vi "time course only.vi"() -> ()   [LabVIEW 2016]
uses:
  <vilib>/Utility/file.llb/Read Delimited Spreadsheet (string).vi
  <vilib>/Analysis/NI_AALBase.lvlib
panel:
  out "Histogram Graph 2":T1(graph)
  out "Histogram Graph":T1(graph)
  in  "Save ?":bool
  in  "∮":dbl=4.0
  in  "BM":dbl=23.16
  in  "smooth line":i32=300
  in  "Next Button":bool
  in  "stop 2":dbl=31894.0
  in  "stop":dbl=31744.0
  in  "start 2":dbl=29984.0
  in  "start":dbl=30134.0
  out "XY Graph 2":cluster{dbl[], dbl[]}[](graph)
  out "appended path":path
  out "Filenames":string[](array[string])
  in  "Path Folder":path
  out "path out":path
  out "# of frames":dbl
  out "aoi count repeat":dbl[](array[numeric])
  out "Tandem Yi position":dbl[](array[numeric])
  out "Tandem Xi position":dbl[](array[numeric])
  out "# of AOIs":dbl
  # "Highlight"
  # "Buffer wash"
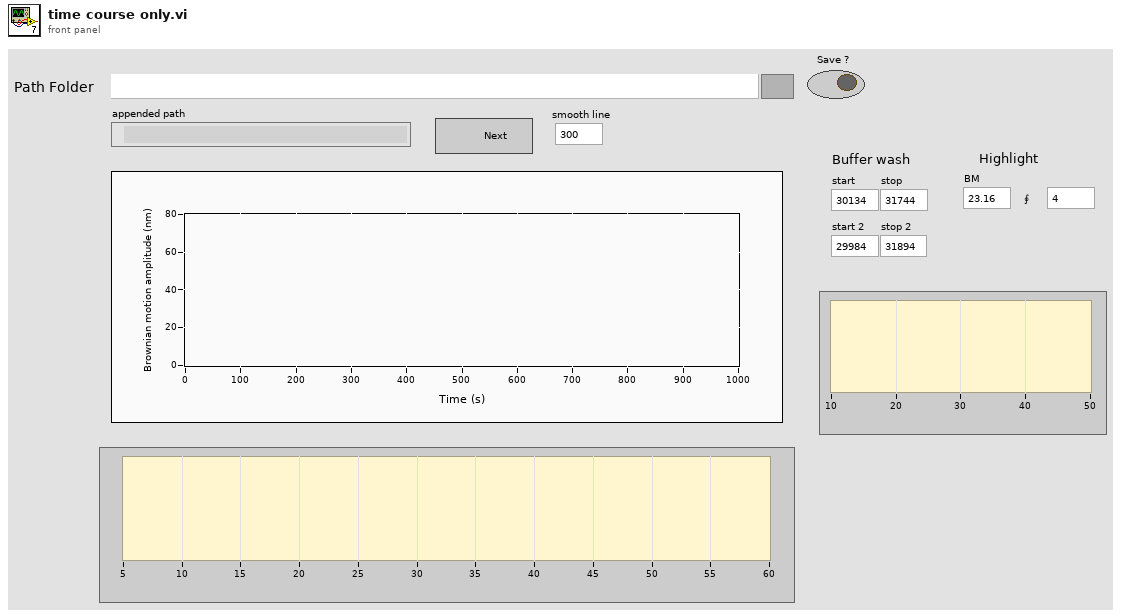
[diagram p1: front panel]
types:
  T1 = cluster{"X Values":dbl[], "Histogram: h(x)":i32[]}
  T2 = typedef "imagedata.ctl" = cluster{"image type":i32, "image depth":i32, "image":u8[], "mask":u8[], "colors":u32[], "Rectangle":cluster{"left":i16, "top":i16, "right":i16, "bottom":i16}}
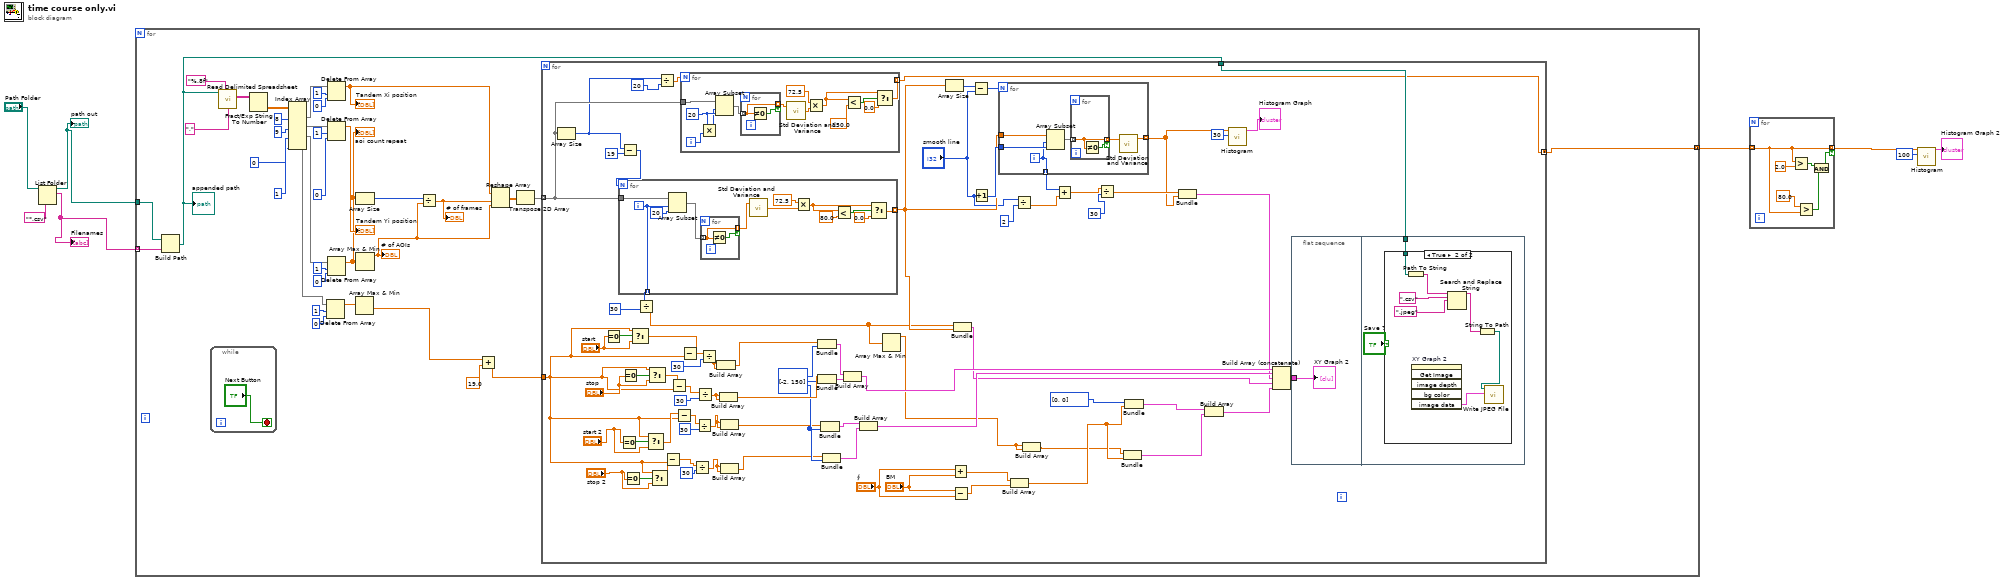
[diagram p0: block diagram]
diagram:
  n1 = List Folder(path="Path Folder", pattern="*.csv") -> (path out=w6:path, filenames=w5:string[])  [unwired: 2 in, 2 out]
  "path out" <- w6
  "Filenames" <- w5
  n2 = for {
    tunnel: w6 -> [w19]
    tunnel: w5 -> [w20] mode=indexing
    tunnel: [w9] -> w2 mode=concatenating
    n3 = Build Path(base path=w19, name or relative path=w20) -> (appended path=w10:path)
    "appended path" <- w10
    n4 = while {
      stop <- "Next Button" stop-if-true
    }
    n5 = call-poly <vilib>:"Read Delimited Spreadsheet.vi"("file path (dialog if empty)"=w10, "format (%s)"="%.8f" ("format (%.3f)"), "delimiter (\\t)"="," ("delimiter (\\t)")) -> ("all rows"=w42:string[][])  [unwired: 7 in, 5 out]
    n6 = Fract/Exp String To Number(string=w42) -> (number=w26:dbl[][])  [unwired: 3 in, 1 out]
    n7 = Index Array(array=w26, index (col) #1=8 ("disabled index (col)"), index (col) #2=9 ("index (col)"), index (col) #3=1 ("index (col)"), index (col) #4=0 ("index (col)")) -> (element #1=w34:dbl[], element #2=w35:dbl[], element #3=w30:dbl[], element #4=w15:dbl[])  [unwired: 4 in]
    n8 = Delete From Array(array=w15, length=1, index=0) -> (array with subset deleted=w14:dbl[])  [unwired: 1 out]
    n9 = Delete From Array(array=w34, length=1, index=0) -> (array with subset deleted=w25:dbl[])  [unwired: 1 out]
    "Tandem Xi position" <- w25
    n10 = Delete From Array(array=w35, length=1, index=0) -> (array with subset deleted=→"Tandem Yi position":dbl[])  [unwired: 1 out]
    n11 = Delete From Array(array=w30, length=1, index=0) -> (array with subset deleted=w28:dbl[])  [unwired: 1 out]
    "aoi count repeat" <- w28
    n12 = Array Max & Min(array=w14) -> (min value=w13:dbl)  [unwired: 3 out]
    n13 = Array Size(array=w28) -> (size(s)=w27:i32)
    n14 = Array Max & Min(array=w28) -> (max value=w23:dbl)  [unwired: 3 out]
    "# of AOIs" <- w23
    n15 = Divide(x=w27, y=w23) -> (x/y=w24:dbl)
    "# of frames" <- w24
    n16 = Add(x=w13, y=19.0) -> (x+y=w12:dbl)
    n17 = Reshape Array(w25, w24, w23) -> (w22:dbl[][])
    n18 = Transpose 2D Array(2D array=w22) -> (transposed array=w21:dbl[][])
    n19 = for {
      tunnel: w21 -> [w51] mode=indexing
      tunnel: w12 -> [w90]
      tunnel: w10 -> [w55]
      tunnel: [w47] -> w9 mode=concatenating
      w109 = i32[] [-2, 150]
      n20 = Array Size(array=w51) -> (size(s)=w49:i32)
      n21 = Equal To 0?(x="start") -> (x = 0?=w102:bool)
      n22 = Equal To 0?(x="start 2") -> (x = 0?=w98:bool)
      n23 = Subtract(x=w49, y=19 ("length")) -> (x-y=w83:i32)
      n24 = for {
        N: w83 -> [_]
        tunnel: w51 -> [w165]
        tunnel: [w157] -> w117 mode=indexing
        tunnel: [w154] -> w116 mode=indexing
        i -> [w154]
        n25 = Array Subset(array=w165, index=w154, length=20) -> (w156:dbl[])
        n26 = for {
          tunnel: w156 -> [w167] mode=indexing
          tunnel: [w167] -> w155 mode=indexing if=w166
          n27 = Not Equal To 0?(x=w167) -> (x != 0?=w166:bool)
        }
        n28 = call <vilib>:"Std Deviation and Variance.vi"("X"=w155) -> ("standard deviation"=w163:dbl)  [unwired: 1 in, 2 out]
        n29 = Multiply(x=72.5, y=w163) -> (x*y=w158:dbl)
        n30 = Less?(x=w158, y=80.0) -> (x < y?=w160:bool)
        n31 = Select(t=w158, s=w160, f=0.0 ("y")) -> (s? t:f=w157:dbl)
      }
      n32 = Equal To 0?(x="stop") -> (x = 0?=w99:bool)
      n33 = Equal To 0?(x="stop 2") -> (x = 0?=w97:bool)
      n34 = Select(t=w90, s=w102, f="start") -> (s? t:f=w101:dbl)
      n35 = Divide(x=w116, y=30 ("length")) -> (x/y=w62:dbl[])
      n36 = Select(t=w90, s=w98, f="start 2") -> (s? t:f=w93:dbl)
      n37 = Select(t=w90, s=w99, f="stop") -> (s? t:f=w96:dbl)
      n38 = Select(t=w90, s=w97, f="stop 2") -> (s? t:f=w91:dbl)
      n39 = Divide(x=w49, y=20 ("length")) -> (x/y=w48:dbl)
      n40 = Subtract(x=w91, y=w90) -> (x-y=w68:dbl)
      n41 = Subtract(x=w96, y=w90) -> (x-y=w75:dbl)
      n42 = Subtract(x=w93, y=w90) -> (x-y=w71:dbl)
      n43 = for {
        N: w48 -> [_]
        tunnel: w51 -> [w133]
        tunnel: [w121] -> w47 mode=indexing
        i -> [w131]
        w132 = 20 ("length")
        n44 = Multiply(x=w132, y=w131) -> (x*y=w130:i32)
        n45 = Array Subset(array=w133, index=w130, length=w132) -> (w129:dbl[])
        n46 = for {
          tunnel: w129 -> [w135] mode=indexing
          tunnel: [w135] -> w128 mode=indexing if=w134
          n47 = Not Equal To 0?(x=w135) -> (x != 0?=w134:bool)
        }
        n48 = call <vilib>:"Std Deviation and Variance.vi"("X"=w128) -> ("standard deviation"=w127:dbl)  [unwired: 1 in, 2 out]
        n49 = Multiply(x=72.5, y=w127) -> (x*y=w122:dbl)
        n50 = Less?(x=w122, y=150.0) -> (x < y?=w124:bool)
        n51 = Select(t=w122, s=w124, f=0.0 ("y")) -> (s? t:f=w121:dbl)
      }
      n52 = Subtract(x=w101, y=w90) -> (x-y=w103:dbl)
      n53 = Divide(x=w68, y=30 ("length")) -> (x/y=w67:dbl)
      n54 = Divide(x=w71, y=30 ("length")) -> (x/y=w70:dbl)
      n55 = Divide(x=w75, y=30 ("length")) -> (x/y=w74:dbl)
      n56 = Divide(x=w103, y=30 ("length")) -> (x/y=w77:dbl)
      n57 = Build Array(w77, w77) -> (w111:dbl[])
      n58 = Build Array(w74, w74) -> (w110:dbl[])
      n59 = Build Array(w70, w70) -> (w106:dbl[])
      n60 = Build Array(w67, w67) -> (w105:dbl[])
      n61 = Bundle(w111, w109) -> (w114:cluster{dbl[], i32[]})  [unwired: 1 in]
      n62 = Bundle(w110, w109) -> (w115:cluster{dbl[], i32[]})  [unwired: 1 in]
      n63 = Bundle(w106, w109) -> (w108:cluster{dbl[], i32[]})  [unwired: 1 in]
      n64 = Bundle(w105, w109) -> (w107:cluster{dbl[], i32[]})  [unwired: 1 in]
      n65 = Build Array(w114, w115) -> (w112:cluster{dbl[], i32[]}[])
      n66 = Build Array(w108, w107) -> (w104:cluster{dbl[], i32[]}[])
      n67 = Array Max & Min(array=w62) -> (max value=w61:dbl)  [unwired: 3 out]
      n68 = Array Size(array=w117) -> (size(s)=w118:i32)
      n69 = Add(x="∮", y="BM") -> (x+y=w58:dbl)
      n70 = Subtract(x="BM", y="∮") -> (x-y=w57:dbl)
      n71 = Bundle(w62, w117) -> (w88:cluster{dbl[], dbl[]})  [unwired: 1 in]
      n72 = Subtract(x=w118, y="smooth line") -> (x-y=w119:i32)
      n73 = Increment(x="smooth line") -> (x+1=w120:i32)
      n74 = for {
        N: w119 -> [_]
        tunnel: w117 -> [w151]
        tunnel: [w148] -> w52 mode=indexing
        tunnel: w120 -> [w147]
        tunnel: [w146] -> w89 mode=indexing
        i -> [w146]
        n75 = Array Subset(array=w151, index=w146, length=w147) -> (w150:dbl[])
        n76 = for {
          tunnel: [w152] -> w149 mode=indexing if=w153
          tunnel: w150 -> [w152] mode=indexing
          n77 = Not Equal To 0?(x=w152) -> (x != 0?=w153:bool)
        }
        n78 = call <vilib>:"Std Deviation and Variance.vi"("X"=w149) -> ("mean"=w148:dbl)  [unwired: 1 in, 2 out]
      }
      n79 = Build Array(w58, w57) -> (w56:dbl[])
      n80 = Divide(x="smooth line", y=2) -> (x/y=w86:dbl)
      n81 = Build Array(w61, w61) -> (w46:dbl[])
      n82 = Add(x=w89, y=w86) -> (x+y=w79:dbl[])
      n83 = Divide(x=w79, y=30 ("length")) -> (x/y=w80:dbl[])
      n84 = Bundle(w46, w56) -> (w66:cluster{dbl[], dbl[]})  [unwired: 1 in]
      n85 = Bundle(i32[] [0, 0], w56) -> (w65:cluster{i32[], dbl[]})  [unwired: 1 in]
      n86 = Bundle(w80, w52) -> (w87:cluster{dbl[], dbl[]})  [unwired: 1 in]
      n87 = Build Array(w65, w66) -> (w63:cluster{dbl[], dbl[]}[])
      n88 = call <vilib>:"Histogram.vi"("intervals"=30, "X"=w52) -> ("Histogram Graph"=→"Histogram Graph":T1)  [unwired: 6 in, 3 out]
      n89 = Build Array (concatenate)(w112, w104, w87, w88, w63) -> (w113:cluster{dbl[], dbl[]}[])
      n90 = flat-sequence {
        tunnel: w113 -> [w136]
        tunnel: w55 -> [w138]
        frame #0 {
          "XY Graph 2" <- w136
        }
        frame #1 {
          n91 = case shown="True" "Save ?" {
            tunnel: w138 -> [_ w144]
            frame False {
            }
            frame True {
              n92 = Path To String(path=w144) -> (string=w143:string)
              n93 = invoke on="XY Graph 2" class="XYGraph (strict)" method="Get Image"() -> ("image data"=w145:T2)  [unwired: 6 in, 5 out]
              n94 = Search and Replace String(input string=w143, search string=".csv", replace string=".jpeg" ("search string")) -> (result string=w140:string)  [unwired: 5 in, 3 out]
              n95 = String To Path(string=w140) -> (path=w139:path)
              n96 = call <vilib>:"Write JPEG File.vi"("image data"=w145, "path to JPEG file"=w139) -> ()  [unwired: 8 in, 2 out]
            }
          }
        }
      }
    }
  }
  n97 = for {
    tunnel: w2 -> [w171] mode=indexing
    tunnel: [w171] -> w1 mode=indexing if=w168
    n98 = Greater?(x=w171, y=2.0) -> (0:w169:bool)
    n99 = Greater?(x=80.0 ("y"), y=w171) -> (0:w170:bool)
    n100 = And(x=w169, y=w170) -> (x .and. y?=w168:bool)
  }
  n101 = call <vilib>:"Histogram.vi"("intervals"=100, "X"=w1) -> ("Histogram Graph"=→"Histogram Graph 2":T1)  [unwired: 6 in, 3 out]
